vi "main.vi"() -> ()   [LabVIEW 2020]
uses:
  controls/target_configuration_cluster.ctl
  controls/state_data_cluster.ctl
  tree_control/vs_tree_control.lvclass
  NationalInstruments.VeriStand.SystemStorage
  NationalInstruments.VeriStand.SystemDefinitionAPI
  <vilib>/addons/VeriStand Custom Device Scripting APIs/Data Sharing Framework/Data Sharing Framework Custom Device Scripting.lvlib
  NationalInstruments.VeriStand.SystemStorageUI
panel:
  in  "Add Target":bool
  in  "Remove Selected":bool
  in  "Load":bool
  in  "Save":bool
  in  "Import":bool
  in  "Export":bool
  in  "SysDef View":refnum<k24>(container)
  out "Target ID":T1
  # "* You must select a target you would like to configure \n   in the SysDef View in order to interact with this pane"
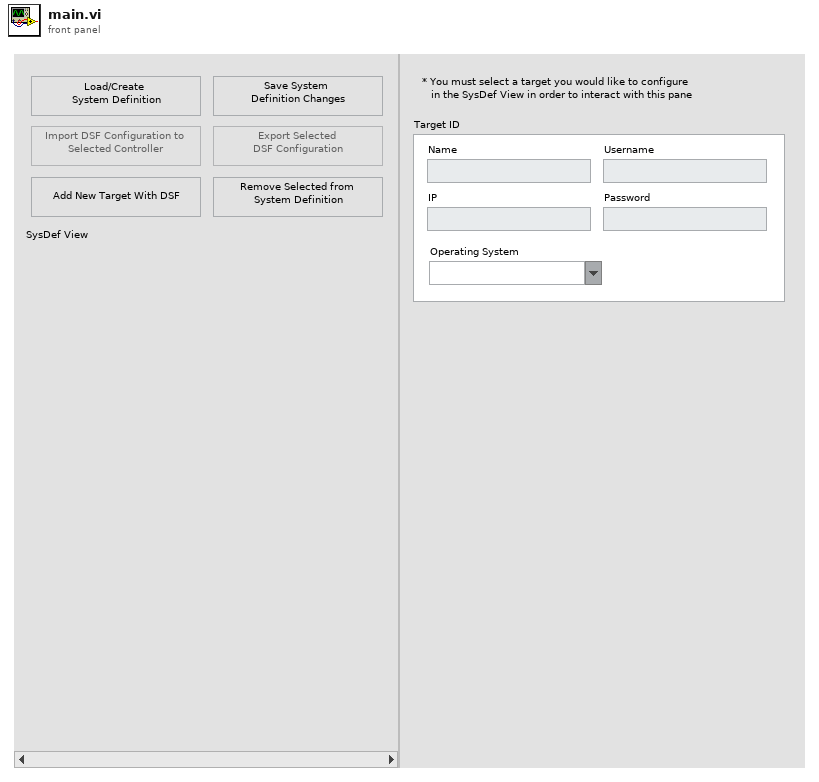
[diagram p1: front panel]
types:
  T1 = typedef "target_configuration_cluster.ctl" = cluster{"Name":string, "IP":string, "Username":string, "Password":string, "Operating System":string}
  T2 = typedef "state_data_cluster.ctl" = cluster{"vsd":refnum<k24>, "vs_tree_control":refnum<class "vs_tree_control.lvclass">}
  T3 = enum8{"Enabled", "Disabled", "Disabled and Grayed Out"}
  T4 = typedef "Custom Device API.lvlib/Custom Device Item Ref.ctl" = u64
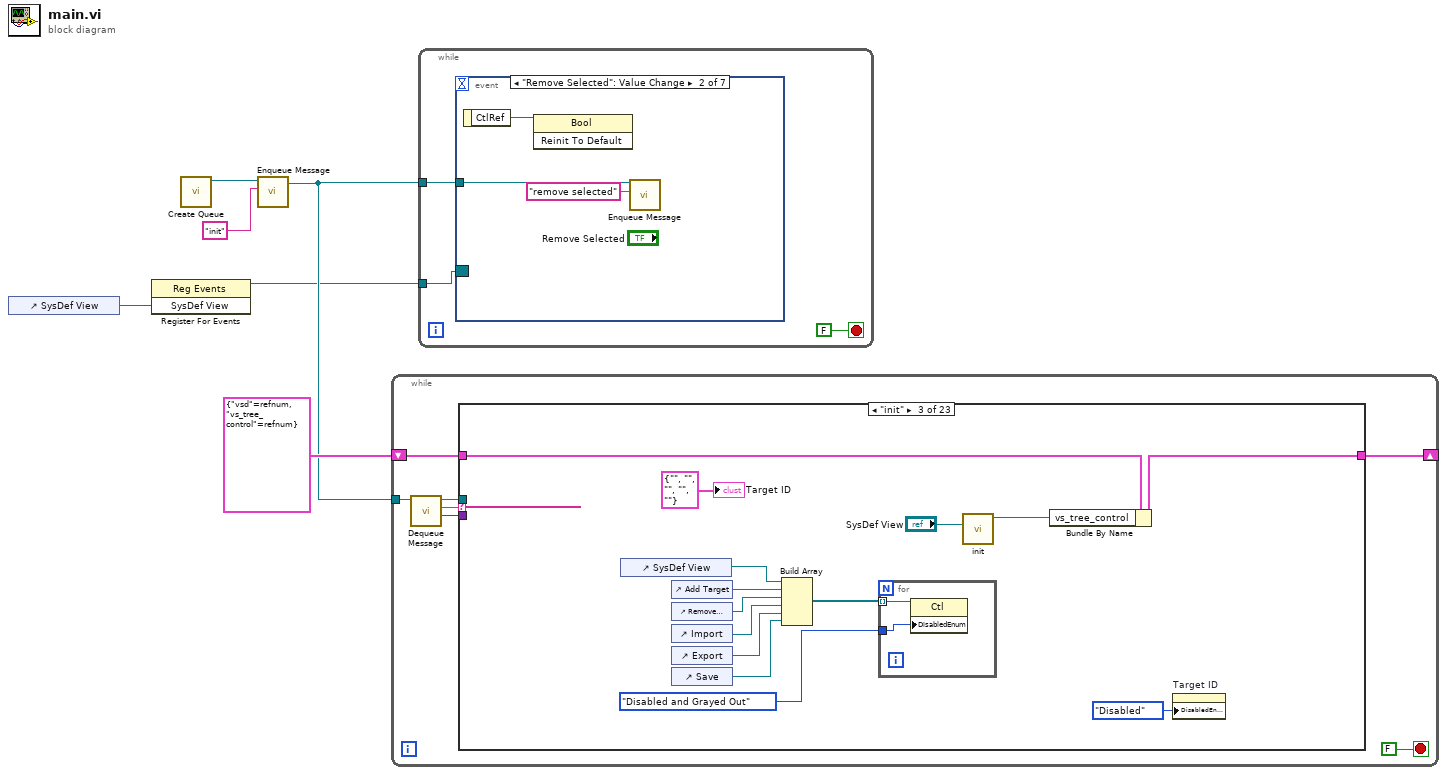
[diagram p0: block diagram]
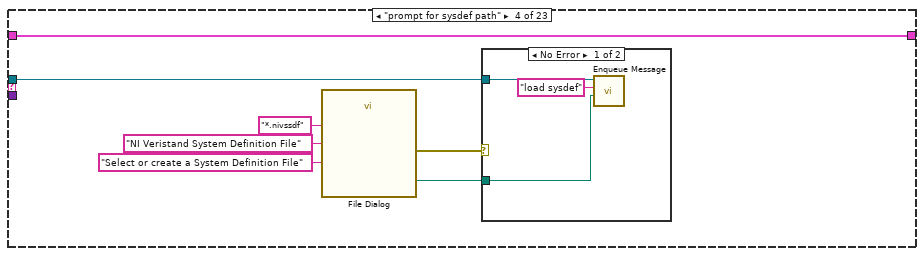
[diagram p4: hidden frame]
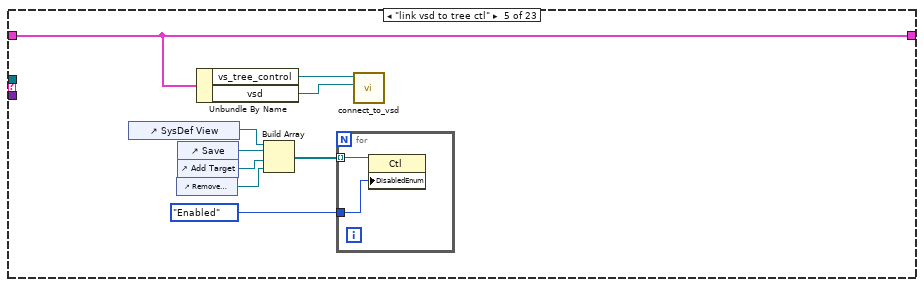
[diagram p6: hidden frame]
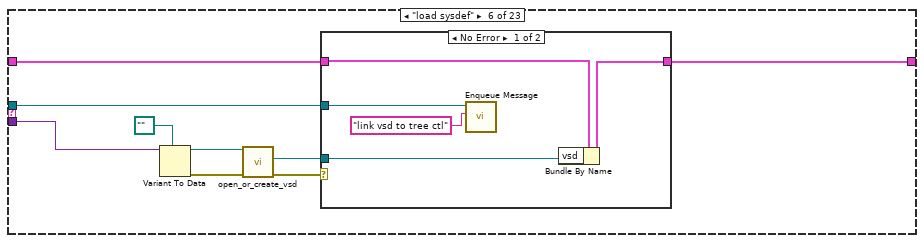
[diagram p7: hidden frame]
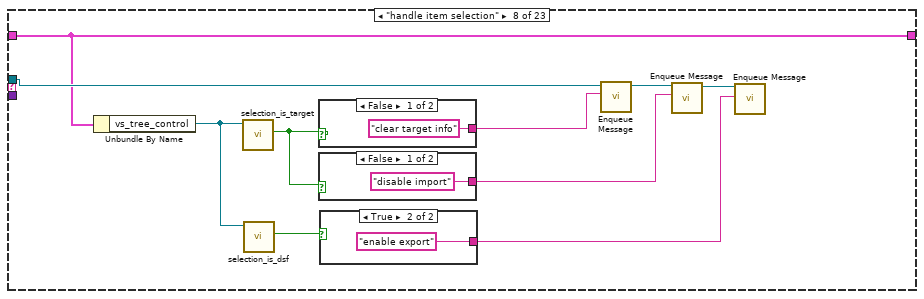
[diagram p10: hidden frame]
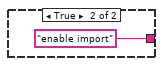
[diagram p11: hidden frame]
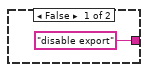
[diagram p12: hidden frame]
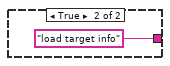
[diagram p13: hidden frame]
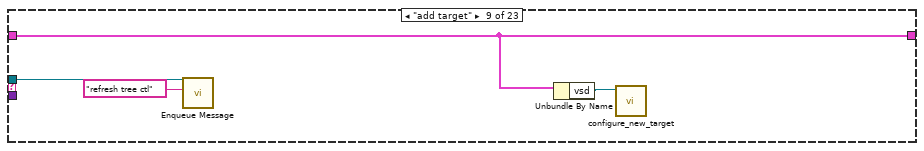
[diagram p14: hidden frame]
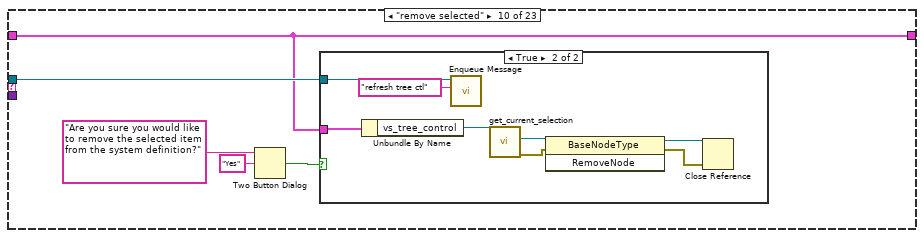
[diagram p15: hidden frame]
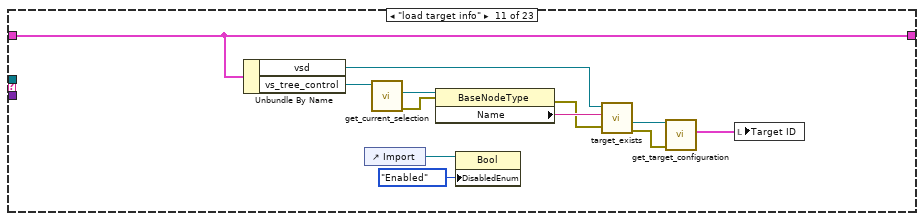
[diagram p17: hidden frame]
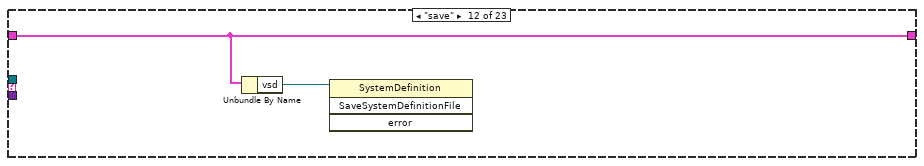
[diagram p18: hidden frame]
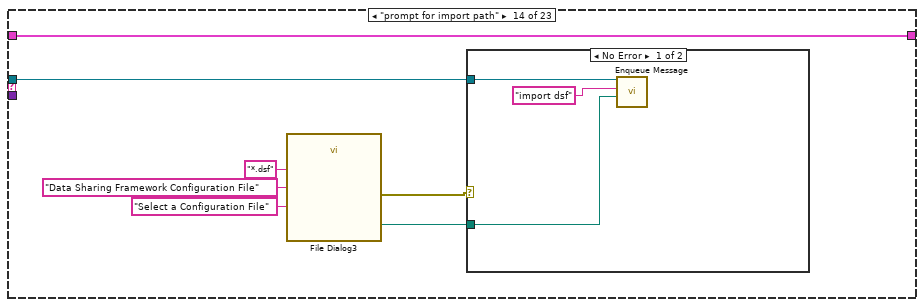
[diagram p20: hidden frame]
diagram:
  n1 = control-ref of="SysDef View"() -> (w2:refnum<vi>)
  n2 = register-events(w2) -> (reference out=w1:refnum<event-registration>)  [unwired: 2 in, 1 out]
  n3 = call "Create Queue.vi"() -> ("Message Queue Out"=w4:refnum<queue>)  [unwired: 10 in, 1 out]
  n4 = call "Enqueue Message.vi"("Message"="init", "Message Queue"=w4) -> ("dup Message Queue"=w3:refnum<queue>)  [unwired: 8 in, 1 out]
  n5 = while {
    tunnel: w3 -> [w11]
    shift-right: [w8] -> _
    shift-left: T2 {"vsd"=refnum, "vs_tree_control"=refnum} -> [w7]
    stop <- FALSE stop-if-true
    n6 = call "Dequeue Message.vi"("Message Queue"=w11) -> ("Message Data"=w9:variant, "Message"=w12:string, "dup Message Queue"=w10:refnum<queue>)  [unwired: 7 in, 1 out]
    n7 = case shown="\"init\"" w12 {
      tunnel: w10 -> [_ _ _ w35 _ w53 _ w77 w86 w93 _ _ _ w118 w136 _ _ _ _ _ _ _ _]
      tunnel: w9 -> [_ _ _ _ _ w61 _ _ _ _ _ _ _ _ w149 _ _ _ _ _ _ _ _]
      tunnel: [w14 w15 w28 w32 w50 w55 w68 w72 w88 w92 w113 w114 w116 w123 w140 w160 w173 w175 w177 w179 w181 w183 w185] -> w8
      tunnel: w7 -> [w14 w15 w29 w32 w50 w54 w68 w72 w88 w92 w113 w114 w116 w123 w140 w160 w173 w175 w177 w179 w181 w183 w185]
      frame Default {
      }
      frame "----- setup -----" {
      }
      frame "init" {
        n8 = control-ref of="SysDef View"() -> (w18:refnum<vi>)
        n9 = control-ref of="Add Target"() -> (w25:refnum<vi>)
        n10 = control-ref of="Remove Selected"() -> (w24:refnum<vi>)
        n11 = control-ref of="Import"() -> (w23:refnum<vi>)
        n12 = control-ref of="Export"() -> (w22:refnum<vi>)
        n13 = control-ref of="Save"() -> (w21:refnum<vi>)
        n14 = Build Array(w18, w25, w24, w23, w22, w21) -> (w20:refnum<vi>[])
        n15 = for {
          tunnel: w20 -> [w31] mode=indexing
          tunnel: T3."Disabled and Grayed Out" ("Disabled") -> [w30]
          n16 = property class="Ctl"(reference=w31, "DisabledEnum"=w30) -> ()  [unwired: 1 in, 2 out]
        }
        n17 = call "init.vi"("tree control reference"="SysDef View") -> ("tree_control out"=w27:refnum<class "vs_tree_control.lvclass">)  [unwired: 9 in, 1 out]
        n18 = Bundle By Name(cluster=w29, "vs_tree_control"=w27) -> (w28:T2)
        n19 = property on="Target ID" class="Clust (strict)"("DisabledEnum"=T3."Disabled" ("Disabled")) -> ()  [unwired: 2 in, 2 out]
        "Target ID" <- T1 {"Name"="", "IP"="", "Username"="", "Password"="", "Operating System"=""} ("Target ID")
      }
      frame "prompt for sysdef path" {
        n20 = call "File Dialog"("prompt"="Select or create a System Definition File", "pattern (all files)"="*.nivssdf" ("pattern label"), "pattern label"="NI Veristand System Definition File") -> ("selected path"=w33:path, "error out"=w34:errorcluster)  [unwired: 9 in, 2 out]
        n21 = case shown="No Error" w34 {
          tunnel: w35 -> [w41 _]
          tunnel: w33 -> [w39 _]
          frame No Error {
            n22 = call "Enqueue Message.vi"("Data"=w39, "Message"="load sysdef", "Message Queue"=w41) -> ()  [unwired: 7 in, 2 out]
          }
          frame Error {
          }
        }
      }
      frame "link vsd to tree ctl" {
        n23 = control-ref of="SysDef View"() -> (w46:refnum<vi>)
        n24 = control-ref of="Remove Selected"() -> (w42:refnum<vi>)
        n25 = control-ref of="Save"() -> (w44:refnum<vi>)
        n26 = control-ref of="Add Target"() -> (w43:refnum<vi>)
        n27 = Unbundle By Name(w50) -> ("vs_tree_control"=w49:refnum<class "vs_tree_control.lvclass">, "vsd"=w48:refnum<k24>)
        n28 = Build Array(w46, w44, w43, w42) -> (w47:refnum<vi>[])
        n29 = for {
          tunnel: w47 -> [w52] mode=indexing
          tunnel: T3."Enabled" ("Disabled") -> [w51]
          n30 = property class="Ctl"(reference=w52, "DisabledEnum"=w51) -> ()  [unwired: 1 in, 2 out]
        }
        n31 = call "connect_to_vsd.vi"("vsd"=w48, "vs_tree_control in"=w49) -> ()  [unwired: 8 in, 2 out]
      }
      frame "load sysdef" {
        n32 = Variant To Data(type=path "", Variant=w61) -> (data=w59:path, error out=w58:errorcluster)  [unwired: 1 in]
        n33 = call "open_or_create_vsd.vi"("error in"=w58, "vsd filepath"=w59) -> ("error out"=w57:errorcluster, "vsd reference"=w56:refnum<k24>)  [unwired: 7 in, 1 out]
        n34 = case shown="No Error" w57 {
          tunnel: w56 -> [w64 _]
          tunnel: [w62 w67] -> w55
          tunnel: w54 -> [w63 w67]
          tunnel: w53 -> [w66 _]
          frame No Error {
            n35 = call "Enqueue Message.vi"("Message"="link vsd to tree ctl", "Message Queue"=w66) -> ()  [unwired: 8 in, 2 out]
            n36 = Bundle By Name(cluster=w63, "vsd"=w64) -> (w62:T2)
          }
          frame Error {
          }
        }
      }
      frame "----- General -----" {
      }
      frame "handle item selection" {
        n37 = Unbundle By Name(w72) -> ("vs_tree_control"=w73:refnum<class "vs_tree_control.lvclass">)
        n38 = call "selection_is_target.vi"("vs_tree_control in"=w73) -> ("is target?"=w71:bool)  [unwired: 8 in, 2 out]
        n39 = call "selection_is_dsf.vi"("vs_tree_control in"=w73) -> ("is dsf?"=w76:bool)  [unwired: 8 in, 2 out]
        n40 = case shown="False" w71 {
          tunnel: ["clear target info" ("Message") "load target info" ("Message")] -> w78
          frame False {
          }
          frame True {
          }
        }
        n41 = case shown="False" w71 {
          tunnel: ["disable import" ("Message") "enable import" ("Message")] -> w74
          frame False {
          }
          frame True {
          }
        }
        n42 = case shown="True" w76 {
          tunnel: ["disable export" ("Message") "enable export" ("Message")] -> w70
          frame False {
          }
          frame True {
          }
        }
        n43 = call "Enqueue Message.vi"("Message"=w78, "Message Queue"=w77) -> ("dup Message Queue"=w75:refnum<queue>)  [unwired: 8 in, 1 out]
        n44 = call "Enqueue Message.vi"("Message"=w74, "Message Queue"=w75) -> ("dup Message Queue"=w69:refnum<queue>)  [unwired: 8 in, 1 out]
        n45 = call "Enqueue Message.vi"("Message"=w70, "Message Queue"=w69) -> ()  [unwired: 8 in, 2 out]
      }
      frame "add target" {
        n46 = call "Enqueue Message.vi"("Message"="refresh tree ctl", "Message Queue"=w86) -> ()  [unwired: 8 in, 2 out]
        n47 = Unbundle By Name(w88) -> ("vsd"=w85:refnum<k24>)
        n48 = call "configure_new_target.vi"("vsd"=w85) -> ()  [unwired: 11 in]
      }
      frame "remove selected" {
        n49 = Two Button Dialog(message="Are you sure you would like to remove the selected item from the system definition?" ("format string"), 2:"Yes" ("T button name (\"OK\")")) -> (T button?=w90:bool)  [unwired: 1 in]
        n50 = case shown="True" w90 {
          tunnel: w93 -> [_ w100]
          tunnel: w92 -> [_ w99]
          frame False {
          }
          frame True {
            n51 = Unbundle By Name(w99) -> ("vs_tree_control"=w98:refnum<class "vs_tree_control.lvclass">)
            n52 = call "Enqueue Message.vi"("Message"="refresh tree ctl", "Message Queue"=w100) -> ()  [unwired: 8 in, 2 out]
            n53 = call "get_current_selection.vi"("vs_tree_control in"=w98) -> ("error out"=w94:errorcluster, "Selection Reference"=w97:refnum<k24>)  [unwired: 6 in, 3 out]
            n54 = invoke class="BaseNodeType" method="RemoveNode"(reference=w97, error in=w94) -> (reference out=w96:refnum<k24>, error out=w95:errorcluster)  [unwired: 1 in, 1 out]
            n55 = Close Reference(reference=w96, error in (no error)=w95) -> ()  [unwired: 1 out]
          }
        }
      }
      frame "load target info" {
        n56 = Unbundle By Name(w113) -> ("vsd"=w107:refnum<k24>, "vs_tree_control"=w112:refnum<class "vs_tree_control.lvclass">)
        n57 = control-ref of="Import"() -> (w103:refnum<vi>)
        n58 = call "get_current_selection.vi"("vs_tree_control in"=w112) -> ("error out"=w110:errorcluster, "Selection Reference"=w111:refnum<k24>)  [unwired: 6 in, 3 out]
        n59 = property class="BaseNodeType"(reference=w111, error in=w110) -> (error out=w108:errorcluster, "Name"=w109:string)  [unwired: 1 out]
        n60 = property class="Bool"(reference=w103, "DisabledEnum"=T3."Enabled" ("Disabled")) -> ()  [unwired: 1 in, 2 out]
        n61 = call "target_exists.vi"("error in"=w108, "Target Name"=w109, "vsd reference"=w107) -> ("error out"=w104:errorcluster, "target if exists"=w106:refnum<k24>)  [unwired: 5 in, 2 out]
        n62 = call "get_target_configuration.vi"("error in"=w104, "target ref"=w106) -> ("Target Configuration Data"=w105:T1)  [unwired: 7 in, 2 out]
        n63 = local write "Target ID"(w105) -> ()
      }
      frame "save" {
        n64 = Unbundle By Name(w114) -> ("vsd"=w115:refnum<k24>)
        n65 = invoke class="SystemDefinition" method="SaveSystemDefinitionFile"(reference=w115) -> ()  [unwired: 3 in, 4 out]
      }
      frame "-----DSF IO -----" {
      }
      frame "prompt for import path" {
        n66 = call "File Dialog3"("prompt"="Select a Configuration File", "pattern (all files)"="*.dsf" ("pattern label"), "pattern label"="Data Sharing Framework Configuration File") -> ("selected path"=w117:path, "error out"=w119:errorcluster)  [unwired: 9 in, 2 out]
        n67 = case shown="No Error" w119 {
          tunnel: w118 -> [w126 _]
          tunnel: w117 -> [w125 _]
          frame No Error {
            n68 = call "Enqueue Message.vi"("Data"=w125, "Message"="import dsf", "Message Queue"=w126) -> ()  [unwired: 7 in, 2 out]
          }
          frame Error {
          }
        }
      }
      frame "import dsf" {
        w145 = refnum<k24> refnum  # target class
        n69 = Variant To Data(type=path "", Variant=w149) -> (data=w141:path, error out=w142:errorcluster)  [unwired: 1 in]
        n70 = Unbundle By Name(w140) -> ("vs_tree_control"=w147:refnum<class "vs_tree_control.lvclass">)
        n71 = call "fetch_selection_node_reference.vi"("error in"=w142, "vs_tree_control in"=w147) -> ("error out"=w144:errorcluster, "Selected Node"=w146:refnum<k24>)  [unwired: 7 in, 1 out]
        n72 = To More Specific Class(target class=w145, reference=w146, error in=w144) -> (specific class reference=w130:refnum<k24>, error out=w129:errorcluster)
        n73 = call <vilib>:"Find.vi"("error in"=w129, "target in"=w130) -> ("error out"=w133:errorcluster, "data sharing framework custom device"=w134:T4, "target out"=w131:refnum<k24>, "found?"=w132:bool)  [unwired: 6 in]
        n74 = case shown="True" w132 {
          tunnel: w134 -> [_ w155]
          tunnel: w133 -> [w151 w154]
          tunnel: [w151 w153] -> w127
          tunnel: w131 -> [w150 w152]
          tunnel: [w150 w152] -> w128
          frame False {
          }
          frame True {
            n75 = call <vilib>:"Remove.vi"("error in"=w154, "data sharing framework custom device"=w155) -> ("error out"=w153:errorcluster)  [unwired: 9 in]
          }
        }
        n76 = call "Enqueue Message.vi"("Message"="refresh tree ctl", "Message Queue"=w136) -> ()  [unwired: 8 in, 2 out]
        n77 = call "fetch_or_create_dsf.vi"("error in"=w127, "target in"=w128) -> ("error out"=w139:errorcluster, "dsf id"=w135:T4, "target out"=w138:refnum<k24>)  [unwired: 7 in]
        n78 = call <vilib>:"Import Configuration.vi"("error in"=w139, "configuration file path"=w141, "data sharing framework custom device"=w135) -> ("error out"=w143:errorcluster)  [unwired: 7 in, 1 out]
        n79 = Close Reference(reference=w138, error in (no error)=w143) -> ()  [unwired: 1 out]
      }
      frame "export" {
        n80 = Unbundle By Name(w160) -> ("vs_tree_control"=w159:refnum<class "vs_tree_control.lvclass">)
        n81 = call "selection_is_dsf.vi"("vs_tree_control in"=w159) -> ("error out"=w157:errorcluster, "is dsf?"=w158:bool, "vs_tree_control out"=w156:refnum<class "vs_tree_control.lvclass">)  [unwired: 8 in]
        n82 = case shown="True" w158 {
          tunnel: w157 -> [_ w167]
          tunnel: w156 -> [_ w166]
          frame False {
            n83 = One Button Dialog(message="You must first select a DSF item in the VeriStand Tree Control") -> ()  [unwired: 1 in, 1 out]
          }
          frame True {
            n84 = call "File Dialog2"("prompt"="Select or create a Configuration File", "error in"=w167, "pattern (all files)"="*.dsf" ("pattern label"), "pattern label"="Data Sharing Framework Configuration File") -> ("selected path"=w168:path, "error out"=w165:errorcluster)  [unwired: 8 in, 2 out]
            n85 = call "get_current_selection.vi"("error in"=w165, "vs_tree_control in"=w166) -> ("error out"=w163:errorcluster, "Selection ID"=w164:u64, "Selection Reference"=w162:refnum<k24>)  [unwired: 5 in, 2 out]
            n86 = call <vilib>:"Export Configuration.vi"("error in"=w163, "configuration file path"=w168, "data sharing framework custom device"=w164) -> ("error out"=w169:errorcluster)  [unwired: 6 in, 2 out]
            n87 = Close Reference(reference=w162, error in (no error)=w169) -> ()  [unwired: 1 out]
          }
        }
      }
      frame "----- FP Controls Conditioning -----" {
      }
      frame "disable import" {
        n88 = property on="Import" class="Bool"("DisabledEnum"=T3."Disabled and Grayed Out" ("Disabled")) -> ()  [unwired: 2 in, 2 out]
      }
      frame "enable import" {
        n89 = property on="Import" class="Bool"("DisabledEnum"=T3."Enabled" ("Disabled")) -> ()  [unwired: 2 in, 2 out]
      }
      frame "refresh tree ctl" {
        n90 = Unbundle By Name(w179) -> ("vs_tree_control"=w178:refnum<class "vs_tree_control.lvclass">)
        n91 = call "refresh_ui.vi"("vs_tree_control in"=w178) -> ()  [unwired: 9 in, 2 out]
      }
      frame "clear target id" {
        n92 = local write "Target ID"(T1 {"Name"="", "IP"="", "Username"="", "Password"="", "Operating System"=""} ("Target ID")) -> ()
      }
      frame "disable export" {
        n93 = property on="Export" class="Bool"("DisabledEnum"=T3."Disabled and Grayed Out" ("Disabled")) -> ()  [unwired: 2 in, 2 out]
      }
      frame "enable export" {
        n94 = property on="Export" class="Bool"("DisabledEnum"=T3."Enabled" ("Disabled")) -> ()  [unwired: 2 in, 2 out]
      }
    }
  }
  n95 = while {
    tunnel: w3 -> [w187]
    tunnel: w1 -> [w186]
    stop <- FALSE stop-if-true
    n96 = event shown="[1] \"Remove Selected\": Value Change" {
      selector: w186 -> [_ _ _ _ _ _ _]
      dyn-events: _ -> [_ _ _ _ _ _ _]
      timeout: _ -> [_ _ _ _ _ _ _]
      tunnel: w187 -> [w191 w194 w197 w200 w203 w206 w208]
      event "Load": Value Change {
        n97 = event-data() -> ("CtlRef"=w189:refnum<vi>)  [unwired: 1 in]
        n98 = invoke class="Bool" method="Reinit To Default"(reference=w189) -> ()  [unwired: 2 in, 3 out]
        n99 = call "Enqueue Message.vi"("Message"="prompt for sysdef path", "Message Queue"=w191) -> ()  [unwired: 8 in, 2 out]
      }
      event "Remove Selected": Value Change {
        n100 = event-data() -> ("CtlRef"=w192:refnum<vi>)  [unwired: 1 in]
        n101 = invoke class="Bool" method="Reinit To Default"(reference=w192) -> ()  [unwired: 2 in, 3 out]
        n102 = call "Enqueue Message.vi"("Message"="remove selected", "Message Queue"=w194) -> ()  [unwired: 8 in, 2 out]
      }
      event "Export": Value Change {
        n103 = event-data() -> ("CtlRef"=w195:refnum<vi>)  [unwired: 1 in]
        n104 = invoke class="Bool" method="Reinit To Default"(reference=w195) -> ()  [unwired: 2 in, 3 out]
        n105 = call "Enqueue Message.vi"("Message"="export", "Message Queue"=w197) -> ()  [unwired: 8 in, 2 out]
      }
      event "Save": Value Change {
        n106 = event-data() -> ("CtlRef"=w198:refnum<vi>)  [unwired: 1 in]
        n107 = invoke class="Bool" method="Reinit To Default"(reference=w198) -> ()  [unwired: 2 in, 3 out]
        n108 = call "Enqueue Message.vi"("Message"="save", "Message Queue"=w200) -> ()  [unwired: 8 in, 2 out]
      }
      event "Add Target": Value Change {
        n109 = event-data() -> ("CtlRef"=w201:refnum<vi>)  [unwired: 1 in]
        n110 = invoke class="Bool" method="Reinit To Default"(reference=w201) -> ()  [unwired: 2 in, 3 out]
        n111 = call "Enqueue Message.vi"("Message"="add target", "Message Queue"=w203) -> ()  [unwired: 8 in, 2 out]
      }
      event "Import": Value Change {
        n112 = event-data() -> ("CtlRef"=w204:refnum<vi>)  [unwired: 1 in]
        n113 = invoke class="Bool" method="Reinit To Default"(reference=w204) -> ()  [unwired: 2 in, 3 out]
        n114 = call "Enqueue Message.vi"("Message"="prompt for import path", "Message Queue"=w206) -> ()  [unwired: 8 in, 2 out]
      }
      event Mouse Down {
        n115 = event-data() -> ()  [unwired: 1 in, 1 out]
        n116 = call "Enqueue Message.vi"("Message"="handle item selection", "Message Queue"=w208) -> ()  [unwired: 8 in, 2 out]
      }
    }
  }
